vi "Map Channels (Multiple).vi"(8 "error in (no error)":errorcluster, 9 "Destinations":string[](array[string]), 10 "Sources":string[](array[string]), 11 "Loop Data":T1) -> (0 "error out":errorcluster)   [LabVIEW 2016, in "System Mapping Tool.lvlib"]
uses:
  System Mapping Tool.lvlib
  TypeDefs/Loop Data.ctl
  TypeDefs/UI Refs.ctl
  NationalInstruments.VeriStand.SystemDefinitionAPI
  NationalInstruments.VeriStand.SystemStorageUI
  TypeDefs/Mapping Error.ctl
  TypeDefs/Mapping Error Cluster.ctl
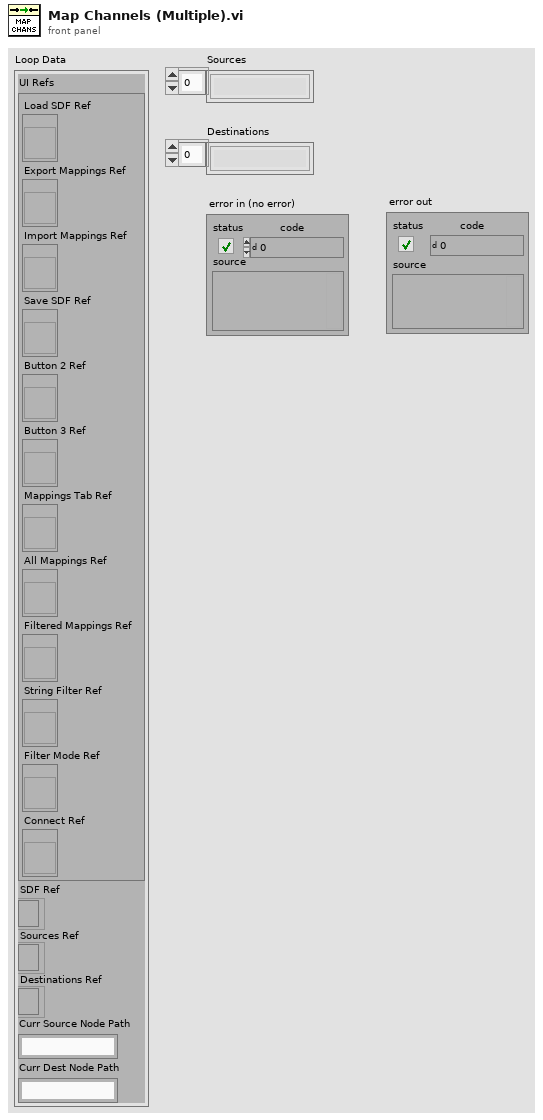
[diagram p1: front panel]
types:
  T1 = typedef "System Mapping Tool.lvlib/Loop Data.ctl" = cluster{"UI Refs":T2, "SDF Ref":refnum<k24>, "Sources Ref":refnum<k24>, "Destinations Ref":refnum<k24>, "Curr Source Node Path":string, "Curr Dest Node Path":string}
  T2 = typedef "System Mapping Tool.lvlib/UI Refs.ctl" = cluster{"Load SDF Ref":refnum<vi>, "Export Mappings Ref":refnum<vi>, "Import Mappings Ref":refnum<vi>, "Save SDF Ref":refnum<vi>, "Button 2 Ref":refnum<vi>, "Button 3 Ref":refnum<vi>, "Mappings Tab Ref":refnum<vi>, "All Mappings Ref":refnum<vi>, "Filtered Mappings Ref":refnum<vi>, "String Filter Ref":refnum<vi>, "Filter Mode Ref":refnum<vi>, "Connect Ref":refnum<vi>}
  T3 = typedef "System Mapping Tool.lvlib/Mapping Error Cluster.ctl" = cluster{"Error?":bool, "Reason":T4, "Source":string, "Destination":string, "Line":i32}
  T4 = typedef "System Mapping Tool.lvlib/Mapping Error.ctl" = enum16{"No error", "Channels already mapped", "Source is not valid", "Destination is not valid", "Destination already mapped", "Destination mapped twice"}
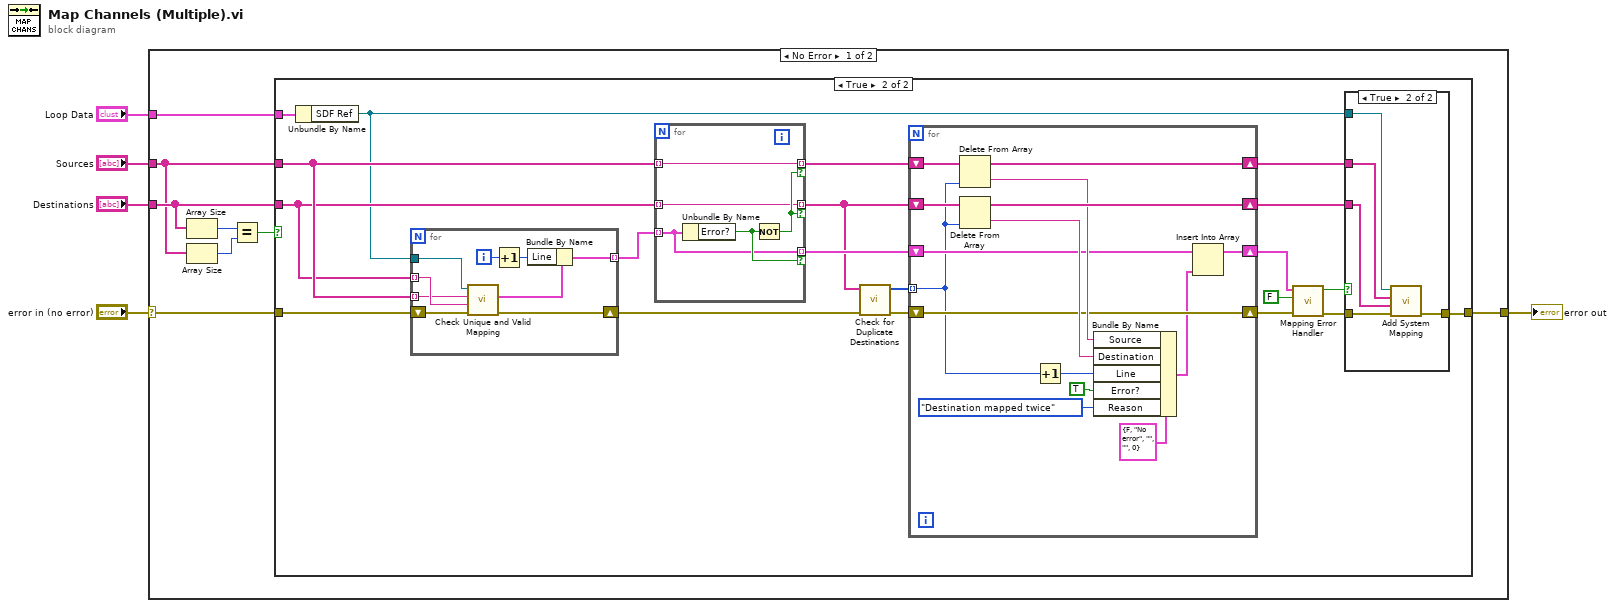
[diagram p0: block diagram]
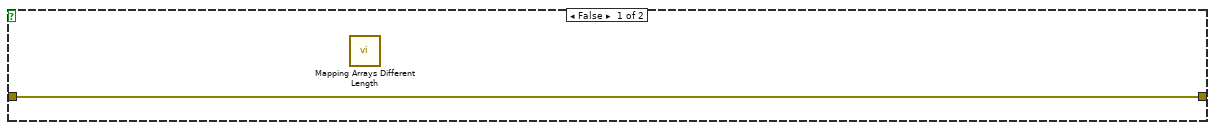
[diagram p2: hidden frame]
diagram:
  n1 = case shown="No Error" "error in (no error)" {
    selector: "error in (no error)" -> [w13 w70]
    tunnel: [w9 w70] -> w4
    tunnel: "Sources" -> [w7 _]
    tunnel: "Destinations" -> [w8 _]
    tunnel: "Loop Data" -> [w6 _]
    frame No Error {
      n2 = Array Size(array=w8) -> (size(s)=w12:i32)
      n3 = Array Size(array=w7) -> (size(s)=w11:i32)
      n4 = Equal?(x=w12, y=w11) -> (x = y?=w10:bool)
      n5 = case shown="True" w10 {
        tunnel: w13 -> [w14 w34]
        tunnel: [w14 w29] -> w9
        tunnel: w7 -> [_ w31]
        tunnel: w8 -> [_ w30]
        tunnel: w6 -> [_ w33]
        frame False {
          n6 = call "Mapping Arrays Different Length.vi"() -> ()  [unwired: 12 in]
        }
        frame True {
          n7 = Unbundle By Name(w33) -> ("SDF Ref"=w16:refnum<k24>)
          n8 = for {
            shift-right: [w66] -> w28
            shift-left: w34 -> [w69]
            tunnel: w30 -> [w68] mode=indexing
            tunnel: w31 -> [w67] mode=indexing
            tunnel: [w63] -> w32 mode=indexing
            tunnel: w16 -> [w65]
            i -> [w62]
            n9 = call "Check Unique and Valid Mapping.vi"("error in (no error)"=w69, "Destination Path"=w68, "Source Path"=w67, "SDF Ref"=w65) -> ("error out"=w66:errorcluster, "Mapping Error"=w64:T3)  [unwired: 6 in]
            n10 = Increment(x=w62) -> (x+1=w61:i32)
            n11 = Bundle By Name(cluster=w64, "Line"=w61) -> (w63:T3)
          }
          n12 = for {
            tunnel: w32 -> [w56] mode=indexing
            tunnel: w31 -> [w59] mode=indexing
            tunnel: w30 -> [w58] mode=indexing
            tunnel: [w59] -> w25 mode=indexing if=w60
            tunnel: [w58] -> w24 mode=indexing if=w60
            tunnel: [w56] -> w26 mode=indexing if=w57
            n13 = Unbundle By Name(w56) -> ("Error?"=w57:bool)
            n14 = Not(x=w57) -> (.not. x?=w60:bool)
          }
          n15 = call "Check for Duplicate Destinations.vi"("error in (no error)"=w28, "Destinations"=w24) -> ("error out"=w27:errorcluster, "Duplicate Indices"=w23:i32[])  [unwired: 8 in]
          n16 = for {
            shift-right: [w48] -> w22
            shift-left: w27 -> [w48]
            shift-right: [w46] -> w20
            shift-left: w26 -> [w47]
            shift-right: [w54] -> w17
            shift-left: w25 -> [w55]
            shift-right: [w52] -> w18
            shift-left: w24 -> [w53]
            tunnel: w23 -> [w41] mode=indexing
            n17 = Delete From Array(array=w55, index=w41) -> (deleted portion=w50:string, array with subset deleted=w54:string[])  [unwired: 1 in]
            n18 = Delete From Array(array=w53, index=w41) -> (deleted portion=w49:string, array with subset deleted=w52:string[])  [unwired: 1 in]
            n19 = Increment(x=w41) -> (x+1=w42:i32)
            n20 = Bundle By Name(cluster=T3 {"Error?"=FALSE, "Reason"=enum."No error", "Source"="", "Destination"="", "Line"=0} ("Mapping Error"), "Source"=w50, "Destination"=w49, "Line"=w42, "Error?"=TRUE, "Reason"=Mapping_Error."Destination mapped twice") -> (w45:T3)
            n21 = Insert Into Array(array=w47, new element=w45) -> (w46:T3[])  [unwired: 1 in]
          }
          n22 = call "Mapping Error Handler.vi"("error in (no error)"=w22, "Single Connect?"=FALSE, "Mapping Errors"=w20) -> ("error out"=w21:errorcluster, "Continue?"=w19:bool)  [unwired: 7 in]
          n23 = case shown="True" w19 {
            tunnel: [w35 w40] -> w29
            tunnel: w21 -> [w35 w39]
            tunnel: w18 -> [_ w37]
            tunnel: w17 -> [_ w36]
            tunnel: w16 -> [_ w38]
            frame False {
            }
            frame True {
              n24 = call "Add System Mapping.vi"("error in (no error)"=w39, "Destinations"=w37, "Sources"=w36, "SDF Ref"=w38) -> ("error out"=w40:errorcluster)  [unwired: 7 in]
            }
          }
        }
      }
    }
    frame Error {
    }
  }
  "error out" <- w4
